vi "GlobalGetAOTFOnOff.vi"() -> ()   [LabVIEW 2013]
panel:
  out "GetAOTF":bool
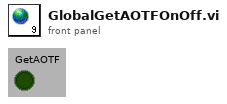
[diagram p1: front panel]
diagram:
